vi "Path-To-Filename-withoutExtension.vi"(0 "Path":path) -> (1 "Fold path":path, 2 "filename without extension":string)   [LabVIEW 2011]
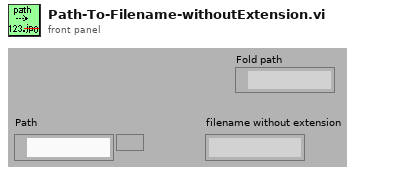
[diagram p1: front panel]
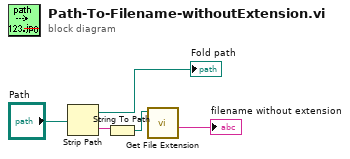
[diagram p0: block diagram]
diagram:
  n1 = Strip Path(path="Path") -> (stripped path=→"Fold path":path, name=w3:string)
  n2 = String To Path(string=w3) -> (path=w4:path)
  n3 = call <vilib>:"Get File Extension.vi"("file"=w4) -> ("filename without extension"=→"filename without extension":string)  [unwired: 1 in, 9 out]
